vi "LED2472G_On LED Matrix.vi"(8 "error in (no error)":errorcluster) -> (0 "error out":errorcluster)   [LabVIEW 2020]
uses:
  <vilib>/MakerHub/LINX/Public/Utilities/Open Local.vi
  <vilib>/MakerHub/LINX/LMH-LINX.lvlib
  RPI_SenseHat/LED2472G/LED2472G/LED2472G.lvclass
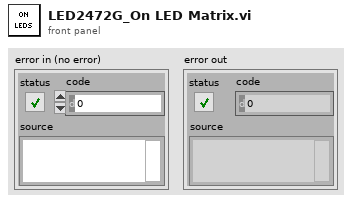
[diagram p1: front panel]
types:
  T1 = typedef "LMH-LINX.lvlib/LINX Ref.ctl" = cluster{"IO":T2, "Interface":T3, "LINX Device Config":T4}
  T2 = typedef "LMH-LINX.lvlib/Platform.ctl" = enum16{"Remote", "Local"}
  T3 = typedef "LMH-LINX.lvlib/Interface.ctl" = enum16{"Serial", "TCP"}
  T4 = typedef "LMH-LINX.lvlib/Device.lvlib/LINX Device Config.ctl" = cluster{"Interface":T3, "COM Port":refnum<visa-resource-name>, "TCP Configuration":T5, "Device Family":u8, "Device ID":u8, "Device Name":string, "TCP Ref":refnum<k5>, "Channels":T6}
  T5 = typedef "LMH-LINX.lvlib/Device.lvlib/TCP Config.ctl" = cluster{"IP Address":string, "Port":u16}
  T6 = typedef "LMH-LINX.lvlib/Channels.ctl" = cluster{"DI":u8[], "DO":u8[], "AI":u8[], "AO":u8[], "PWM":u8[], "QE":u8[], "UART":u8[], "I2C 2":u8[], "SPI":u8[], "CAN":u8[], "Servo":u8[], "AI Ref (V)":dbl, "AI Resolution (Bits)":u8, "AO Ref (V)":dbl, "AO Resolution (Bits)":u8}
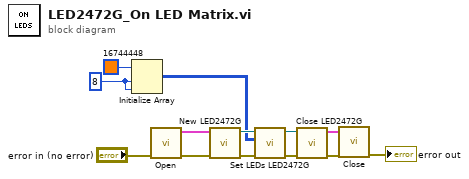
[diagram p0: block diagram]
diagram:
  w2 = 8 ("dimension size")
  n1 = Initialize Array(u32 16744448, w2, w2) -> (w1:u32[][])
  n2 = call-poly <vilib>:"Open.vi"("Error In"="error in (no error)") -> ("Error Out"=w12:errorcluster, "LINX Resource"=w13:T1)  [unwired: 8 in, 1 out]
  n3 = call "New LED2472G.vi"("error in (no error)"=w12, "LINX Resource"=w13) -> ("error out"=w7:errorcluster, "LED2472G out"=w6:refnum<class "LED2472G.lvclass">)  [unwired: 8 in]
  n4 = call "Set LEDs LED2472G.vi"("error in (no error)"=w7, "LED Matrix"=w1, "LED2472G in"=w6) -> ("error out"=w4:errorcluster, "LED2472G out"=w5:refnum<class "LED2472G.lvclass">)  [unwired: 7 in]
  n5 = call "Close LED2472G.vi"("error in (no error)"=w4, "LED2472G in"=w5) -> ("error out"=w11:errorcluster, "LINX Resource"=w10:T1)  [unwired: 8 in]
  n6 = call <vilib>:"Close.vi"("Error In"=w11, "LINX Resource"=w10) -> ("Error Out"=→"error out":errorcluster)  [unwired: 9 in]
